vi "Config Dev Format.vi"(8 "error in":errorcluster, 9 "Loss (0)":i32 min=0 max=4, 10 "Capacitance (0)":i32 min=0 max=4, 11 "VISA resource name":refnum<visa-resource-name>) -> (0 "error out":errorcluster, 3 "VISA resource name out":refnum<visa-resource-name>)   [LabVIEW 2017, in "Andeen-Hagerling 2700.lvlib"]
doc: "This VI sets the deviation format applied to deviation results reported to both the front panel and remote devices."
uses:
  Andeen-Hagerling 2700.lvlib
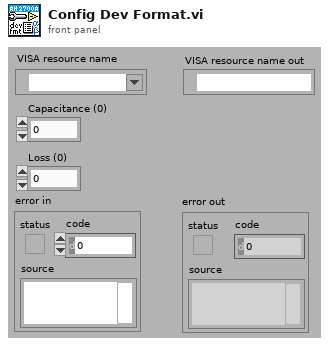
[diagram p1: front panel]
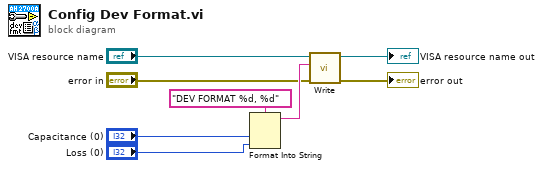
[diagram p0: block diagram]
diagram:
  n1 = Format Into String(format string="DEV FORMAT %d, %d", "Capacitance (0)", "Loss (0)") -> (resulting string=w7:string)  [unwired: 2 in, 1 out]
  n2 = call "Write.vi"("error in"="error in", "command"=w7, "VISA resource name"="VISA resource name") -> ("error out"=→"error out":errorcluster, "VISA resource name out"=→"VISA resource name out":refnum<visa-resource-name>)  [unwired: 7 in]
